vi "能够流畅执行的界面模式.vi"() -> ()   [LabVIEW 2018]
panel:
  out "当前进度":dbl
  out "当前状态":string
  out "滑动杆":u8(slide) scale=0.0..100.0
  in  "下一步":bool
  in  "开始":bool
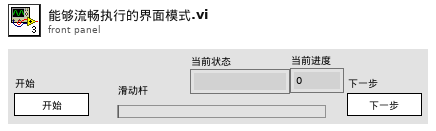
[diagram p1: front panel]
types:
  T1 = enum8{"Enabled", "Disabled", "Disabled and Grayed Out"}
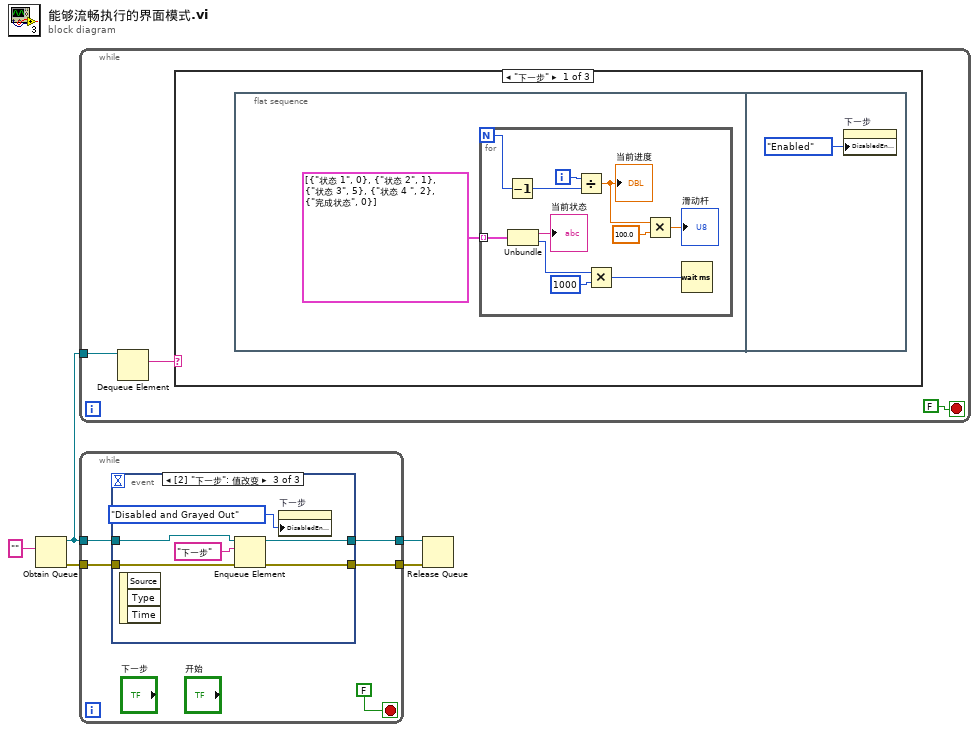
[diagram p0: block diagram]
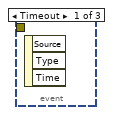
[diagram p4: hidden frame]
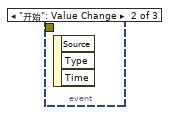
[diagram p5: hidden frame]
diagram:
  n1 = Obtain Queue(element data type="") -> (queue out=w1:refnum<queue>, error out=w4:errorcluster)  [unwired: 4 in, 1 out]
  n2 = while {
    tunnel: w1 -> [w8]
    stop <- FALSE stop-if-true
    n3 = Dequeue Element(queue=w8) -> (element=w6:string)  [unwired: 2 in, 3 out]
    n4 = case shown="\"下一步\"" w6 {
      frame "下一步" {
        n5 = flat-sequence {
          frame #0 {
            n6 = for {
              N -> [w15]
              tunnel: cluster{string, i32}[] [{"状态 1", 0}, {"状态 2", 1}, {"状态 3", 5}, {"状态 4 ", 2}, {"完成状态", 0}] -> [w20] mode=indexing
              i -> [w14]
              n7 = Decrement(x=w15) -> (x-1=w13:i32)
              n8 = Unbundle(w20) -> (→"当前状态":string, w18:i32)
              n9 = Divide(x=w14, y=w13) -> (x/y=w12:dbl)
              "当前进度" <- w12
              n10 = Multiply(x=w18, y=1000) -> (x*y=w19:i32)
              n11 = Multiply(x=w12, y=100.0) -> (x*y=→"滑动杆":dbl)
              n12 = Wait (ms)(milliseconds to wait=w19) -> ()  [unwired: 1 out]
            }
          }
          frame #1 {
            n13 = property on="下一步" class="Bool"("DisabledEnum"=T1."Enabled" ("禁用")) -> ()  [unwired: 2 in, 2 out]
          }
        }
      }
      frame "无错误", Default {
      }
      frame "错误" {
      }
    }
  }
  n14 = while {
    tunnel: w1 -> [w25]
    tunnel: w4 -> [w24]
    tunnel: [w23] -> w3
    tunnel: [w22] -> w2
    stop <- FALSE stop-if-true
    n15 = event shown="[2] \"下一步\": 值改变" {
      selector: _ -> [_ _ _]
      dyn-events: _ -> [_ _ _]
      timeout: _ -> [_ _ _]
      tunnel: w25 -> [_ _ w32]
      tunnel: w24 -> [_ _ w31]
      tunnel: [_ _ w29] -> w23
      tunnel: [_ _ w28] -> w22
      event Timeout {
        n16 = event-data() -> ()  [unwired: 1 in, 3 out]
      }
      event "开始": Value Change {
        n17 = event-data() -> ()  [unwired: 1 in, 3 out]
      }
      event "下一步": Value Change {
        n18 = event-data() -> ()  [unwired: 1 in, 3 out]
        n19 = Enqueue Element(queue=w32, element="下一步" ("元素"), error in (no error)=w31) -> (queue out=w29:refnum<queue>, error out=w28:errorcluster)  [unwired: 1 in, 1 out]
        n20 = property on="下一步" class="Bool"("DisabledEnum"=T1."Disabled and Grayed Out" ("禁用")) -> ()  [unwired: 2 in, 2 out]
      }
    }
  }
  n21 = Release Queue(queue=w3, error in (no error)=w2) -> ()  [unwired: 1 in, 3 out]
